vi "Qbep.vi"(11 "Qbep":dbl) -> (3 "18 punti 1)":T1)   [LabVIEW 2019]
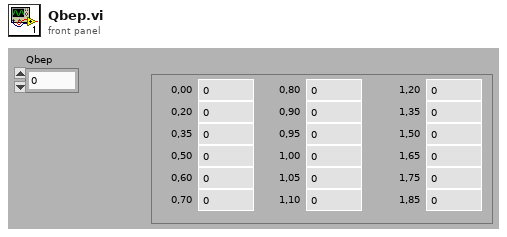
[diagram p1: front panel]
types:
  T1 = cluster{"0,00":dbl, "0,20":dbl, "0,35":dbl, "0,50":dbl, "0,60":dbl, "0,70":dbl, "0,80":dbl, "0,90":dbl, "0,95":dbl, "1,00":dbl, "1,05":dbl, "1,10":dbl, "1,20":dbl, "1,35":dbl, "1,50":dbl, "1,65":dbl, "1,75":dbl, "1,85":dbl}
  T2 = cluster{"[0]":dbl, "[1]":dbl, "[2]":dbl, "[3]":dbl, "[4]":dbl, "[5]":dbl, "[6]":dbl, "[7]":dbl, "[8]":dbl, "[9]":dbl, "[10]":dbl, "[11]":dbl, "[12]":dbl, "[13]":dbl, "[14]":dbl, "[15]":dbl, "[16]":dbl, "[17]":dbl}
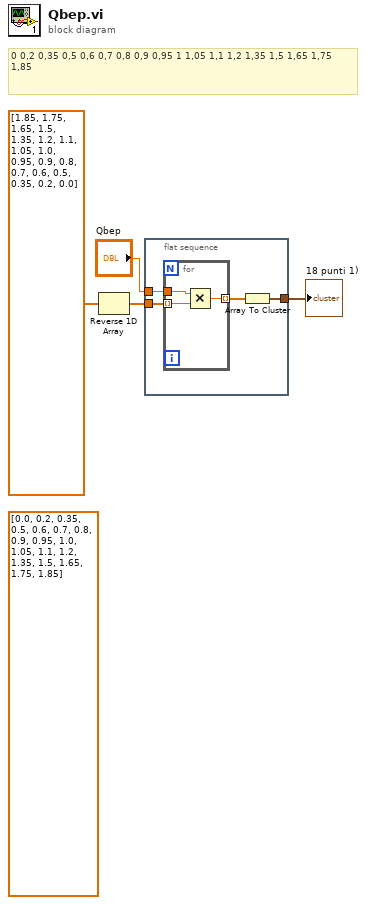
[diagram p0: block diagram]
diagram:
  (unwired) dbl[] [0.0, 0.2, 0.35, 0.5, 0.6, 0.7, 0.8, 0.9, 0.95, 1.0, 1.05, 1.1, 1.2, 1.35, 1.5, 1.65, 1.75, 1.85]
  # "0\t0,2\t0,35\t0,5\t0,6\t0,7\t0,8\t0,9\t0,95\t1\t1,05\t1,1\t1,2\t1,35\t1,5\t1,65\t1,75\t1,85"
  n1 = Reverse 1D Array(array=dbl[] [1.85, 1.75, 1.65, 1.5, 1.35, 1.2, 1.1, 1.05, 1.0, 0.95, 0.9, 0.8, 0.7, 0.6, 0.5, 0.35, 0.2, 0.0] ("array (last n elements first)")) -> (reversed array=w1:dbl[])
  n2 = flat-sequence {
    tunnel: [w7] -> w3
    tunnel: "Qbep" -> [w6]
    tunnel: w1 -> [w5]
    frame #0 {
      n3 = for {
        tunnel: [w11] -> w8 mode=indexing
        tunnel: w6 -> [w10]
        tunnel: w5 -> [w9] mode=indexing
        n4 = Multiply(x=w10, y=w9) -> (x*y=w11:dbl)
      }
      n5 = Array To Cluster(array=w8) -> (cluster=w7:T2)
    }
  }
  "18 punti 1)" <- w3
